vi "vidiff ini section and keys.vi"() -> (1 "DiffArgKeyNames":string[](array[string])=["BD", "FP", "VIattr", "cosmetic"], 2 "Section":string)   [LabVIEW 2016]
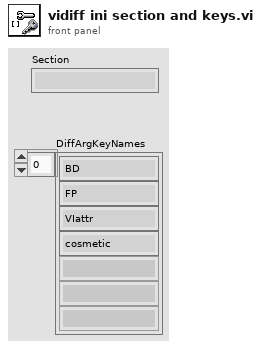
[diagram p1: front panel]
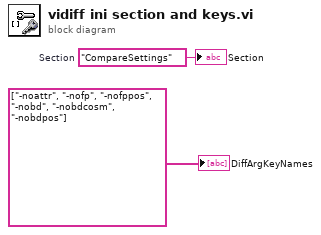
[diagram p0: block diagram]
diagram:
  w2 = "CompareSettings"  # Section
  "DiffArgKeyNames" <- string[] ["-noattr", "-nofp", "-nofppos", "-nobd", "-nobdcosm", "-nobdpos"] ("lv version keys")
  "Section" <- w2
